vi "哪个棋子.vi"(0 "游戏":T1, 1 "X":u8, 2 "Y":u8) -> (3 "棋子类型":enum16{"士兵", "骑士", "主教", "战车", "皇后", "国王", "空"}(ring), 4 "背景颜色":enum16{"白色", "绿色"}(ring), 5 "棋子颜色":enum16{"银色", "黑色"}(ring), 6 "是否为空":bool)   [LabVIEW 2017]
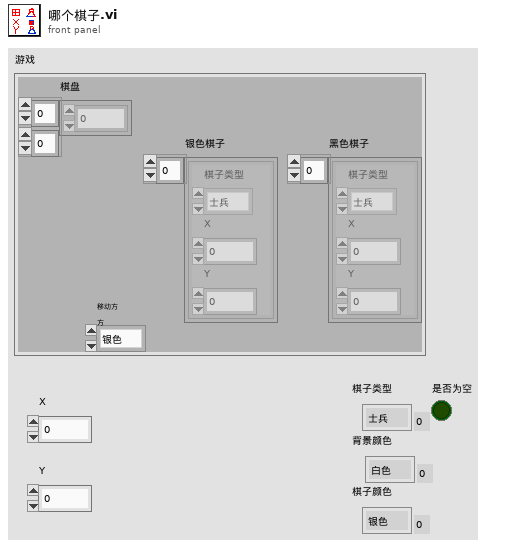
[diagram p1: front panel]
types:
  T1 = cluster{"棋盘":u16[][], "银色棋子":cluster{"棋子类型":enum16{"士兵", "骑士", "主教", "战车", "皇后", "国王", "空"}, "X":u8, "Y":u8}[], "黑色棋子":cluster{"棋子类型":enum16{"士兵", "骑士", "主教", "战车", "皇后", "国王", "空"}, "X":u8, "Y":u8}[], "移动方\n\n方":enum16{"银色", "黑色"}}
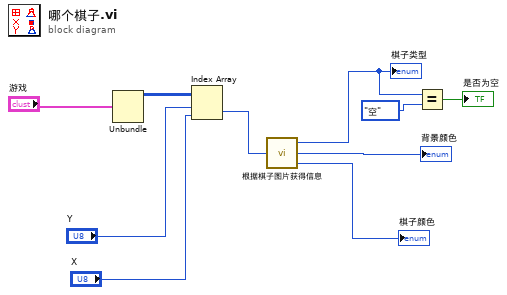
[diagram p0: block diagram]
diagram:
  n1 = Unbundle("游戏") -> ("棋盘"=w10:u16[][])  [unwired: 3 out]
  n2 = Index Array(array=w10, index (row)="Y", index (col)="X") -> (element=w7:u16)
  n3 = call "根据棋子图片获得信息.vi"("棋子"=w7) -> ("棋子类型"=w4:enum16{"士兵", "骑士", "主教", "战车", "皇后", "国王", "空"}, "背景颜色"=→"背景颜色":enum16{"白色", "绿色"}, "棋子颜色"=→"棋子颜色":enum16{"银色", "黑色"})
  "棋子类型" <- w4
  n4 = Equal?(x=w4, y=enum16{"士兵", "骑士", "主教", "战车", "皇后", "国王", "空"}."空") -> (x = y?=→"是否为空":bool)
